vi "HISW_2_PAQ10mil.vi"(8 "error in (no error)":errorcluster, 10 "PAQdatagram IN":T1 {"data" format="%.2f"; "status" format="%08x"}, 11 "AVPP in":refnum<class "AVPP.lvclass">) -> (0 "error out":errorcluster, 3 "AVPP out":refnum<class "AVPP.lvclass">)   [LabVIEW 2014, in "AVPP.lvclass"]
uses:
  AVPP.lvclass
  HISW/controls/typedef_PAQdatagram.ctl
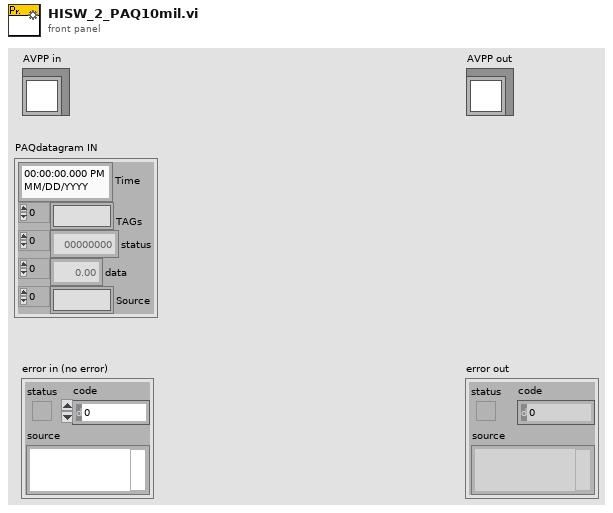
[diagram p1: front panel]
types:
  T1 = typedef "typedef_PAQdatagram.ctl" = cluster{"Time":timestamp, "TAGs":string[], "status":u32[], "data":dbl[], "Source":string[]}
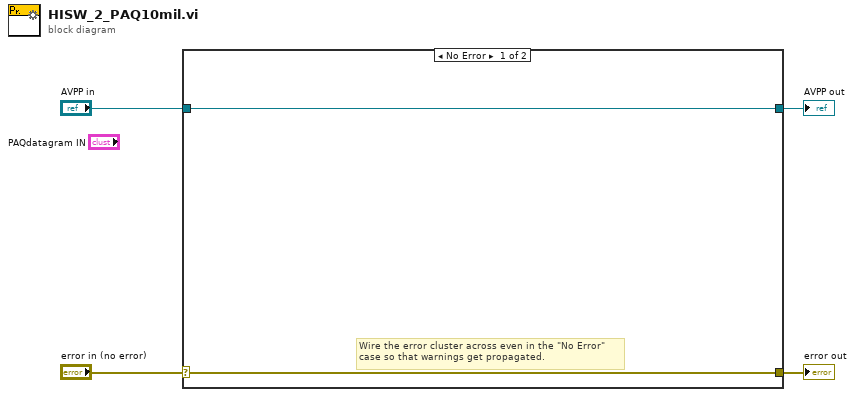
[diagram p0: block diagram]
diagram:
  n1 = case shown="No Error" "error in (no error)" {
    selector: "error in (no error)" -> [w5 w8]
    tunnel: [w5 w8] -> w3
    tunnel: [w6 w7] -> w1
    tunnel: "AVPP in" -> [w6 w7]
    frame No Error {
      # "Wire the error cluster across even in the \"No Error\"\ncase so that warnings get propagated."
    }
    frame Error {
    }
  }
  "error out" <- w3
  "AVPP out" <- w1
